vi "LinearRamp.vi"(8 "Steps":i32, 10 "End Value":dbl, 11 "Start Value":dbl) -> (3 "Ramp Out":dbl[](array[numeric]))   [LabVIEW 2013]
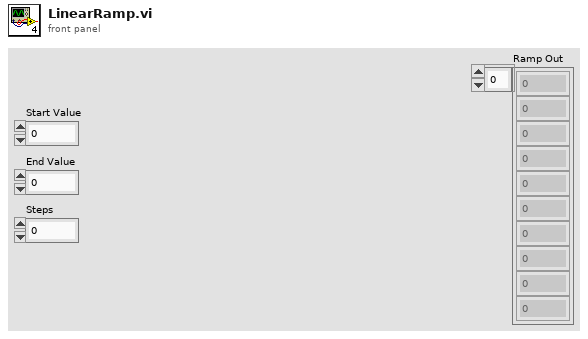
[diagram p1: front panel]
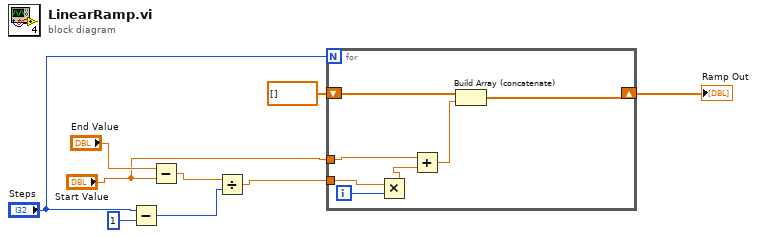
[diagram p0: block diagram]
diagram:
  n1 = Subtract(x="Steps", y=1) -> (x-y=w2:i32)
  n2 = Subtract(x="End Value", y="Start Value") -> (x-y=w8:dbl)
  n3 = Divide(x=w8, y=w2) -> (x/y=w6:dbl)
  n4 = for {
    N: "Steps" -> [_]
    shift-right: [w15] -> w5
    shift-left: dbl[] [] -> [w16]
    tunnel: "Start Value" -> [w14]
    tunnel: w6 -> [w12]
    i -> [w11]
    n5 = Multiply(x=w12, y=w11) -> (x*y=w13:dbl)
    n6 = Add(x=w14, y=w13) -> (x+y=w10:dbl)
    n7 = Build Array (concatenate)(w16, w10) -> (w15:dbl[])
  }
  "Ramp Out" <- w5
